vi "AD7609 global.vi"() -> ()   [LabVIEW 2015]
panel:
  in  "Timeout (ms)":u32=10000
  in  "N channels bytes to read":u8=18
  in  "Sleep state":u8(ring) items=["On", "Standby", "Shutdown"]
  in  "Device serial port":refnum<visa-resource-name>
  in  "Triggering mode":u8(ring) items=["Software", "Hardware"]
  in  "Input voltage range (V)":u8(ring)=1 items=["-5... +5 V", "-10... +10 V"]
  in  "Oversampling ratio":u8(ring) items=["1", "2", "4", "8", "16", "32", "64"]
  in  "Sampling rate (Hz)":sgl=1000.0
  in  "Number of samples":u32=1000
  # "PN 25/11/2014, 17/08/2015,\n23/08/2016"
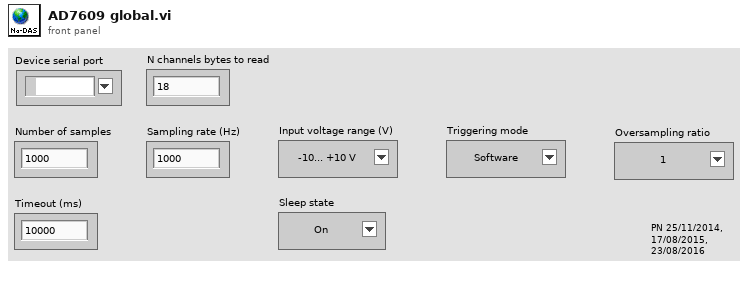
[diagram p1: front panel]
diagram:
